vi "Related Entities.vi"(10 "Conditum:Entity":refnum<class "Entity.lvclass">) -> (1 "error out":errorcluster, 2 "Relations":refnum<class "Entity.lvclass">[](array[class]))   [LabVIEW 2020, in "Conditum.lvlib" / "Entity Manager.lvclass"]
doc: "Given an entity, returns its immediate related entities.\n\nWill return an error if any of the related entities aren't in memory."
uses:
  Entity Manager.lvclass
  Entity Manager.lvclass/Entity Manager.ctl
  Entity/Entity.lvclass
  Columns/Type/Type.lvclass
  Field Type.ctl
  Conditum.lvlib
  Columns/Relation/Relation.lvclass
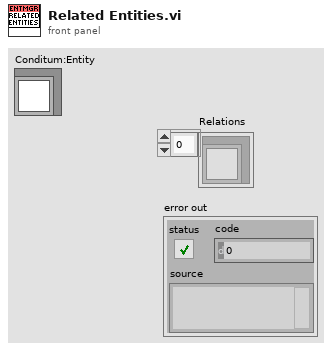
[diagram p1: front panel]
types:
  T1 = typedef "Conditum.lvlib/Field Type.ctl" = enum16{"None", "ID", "Boolean", "Integer", "Double", "Timestamp", "String", "Text", "Entity"}
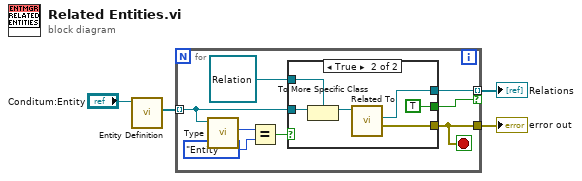
[diagram p0: block diagram]
diagram:
  n1 = call "Entity Definition.vi"("Entity in"="Conditum:Entity") -> ("Definition"=w3:refnum<class "Type.lvclass">[])  [unwired: 10 in]
  n2 = for {
    tunnel: w3 -> [w9] mode=indexing
    tunnel: [w6] -> w2
    tunnel: [w8] -> w1 mode=indexing if=w7
    stop <- w6 stop-if-true
    n3 = call "Type.vi"("Type in"=w9) -> ("Type"=w12:T1)  [unwired: 10 in]
    n4 = Equal?(x=w12, y=Field_Type."Entity") -> (x = y?=w10:bool)
    n5 = case shown="True" w10 {
      tunnel: w9 -> [_ w18]
      tunnel: refnum<class "Relation.lvclass"> refnum ("Conditum:Columns:Relation.lvclass") -> [_ w17]
      tunnel: [_ w15] -> w6
      tunnel: [_ w14] -> w8
      tunnel: [_ TRUE] -> w7
      frame False {
      }
      frame True {
        n6 = To More Specific Class(target class=w17, reference=w18) -> (specific class reference=w16:refnum<class "Relation.lvclass">)  [unwired: 1 in, 1 out]
        n7 = call "Related To.vi"("Relation in"=w16) -> ("error out"=w15:errorcluster, "Related To"=w14:refnum<class "Entity.lvclass">)  [unwired: 9 in]
      }
    }
  }
  "Relations" <- w1
  "error out" <- w2
